vi "Task Init.vi"(8 "error in (no error)":errorcluster, 11 "BasicEventLogger in":refnum<class "BasicEventLogger.lvclass">) -> (0 "error out":errorcluster, 3 "BasicEventLogger out":refnum<class "BasicEventLogger.lvclass">)   [LabVIEW 2020, in "Volatus.lvlib" / "BasicEventLogger.lvclass"]
uses:
  BasicEventLogger.lvclass
  Event.ctl
  Event Level.ctl
  BasicEventLogger.lvclass/BasicEventLogger.ctl
  Volatus.lvlib
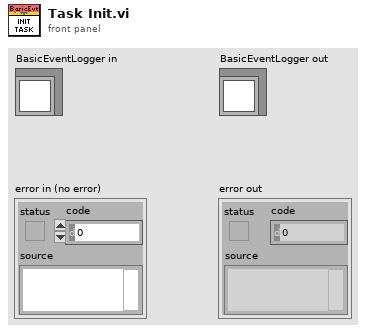
[diagram p1: front panel]
types:
  T1 = typedef "Volatus.lvlib/Event.ctl" = cluster{"Level":T2, "Context":string, "Message":string, "Error":errorcluster}
  T2 = typedef "Volatus.lvlib/Event Level.ctl" = enum16{"Debug", "Info", "Warning", "Error"}
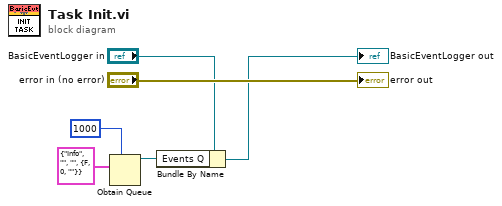
[diagram p0: block diagram]
diagram:
  n1 = Obtain Queue(max queue size (-1, unlimited)=1000, element data type=T1 {"Level"=enum."Info", "Context"="", "Message"="", "Error"={"status"=FALSE, "code"=0, "source"=""}} ("Event")) -> (queue out=w3:refnum<queue>)  [unwired: 3 in, 2 out]
  n2 = Bundle By Name(cluster="BasicEventLogger in", "Events Q"=w3) -> (→"BasicEventLogger out":refnum<class "BasicEventLogger.lvclass">)
  "error out" <- "error in (no error)"
